vi "Convert to Temp (SubVI).vi"(11 "Voltage":fxp<+/-,24,5>) -> (3 "deg C":fxp<+/-,32,13>)   [LabVIEW 2017]
doc: "This VI performs a simple conversion from voltage to degrees celcius."
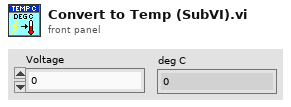
[diagram p1: front panel]
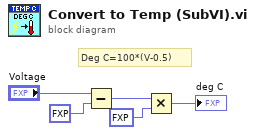
[diagram p0: block diagram]
diagram:
  # "Deg C=100*(V-0.5)"
  n1 = Subtract(x="Voltage", y=fxp<+,1,0> 0.5) -> (x-y=w3:fxp<+/-,25,6>)
  n2 = Multiply(x=w3, y=fxp<+,7,7> 100.0) -> (x*y=→"deg C":fxp<+/-,32,13>)
